vi "Attach Panel Thread.vi"(8 "error in (no error)":errorcluster, 10 "Panel Thread":refnum<class "Panel Controller Interface.lvclass">, 11 "Panel Manager Controller.lvclass":refnum<class "Panel Manager Controller.lvclass">) -> (0 "error out":errorcluster, 3 "Panel Manager Controller.lvclass out":refnum<class "Panel Manager Controller.lvclass">)   [LabVIEW 2015, in "Panel Manager Controller.lvclass"]
uses:
  Panel Manager Controller.lvclass
  _Depences/Panel API/Panel Control_Interface/Panel_interface/Panel Controller Interface.lvclass
  Panel Manager Controller.lvclass/Panel Manager Controller.ctl
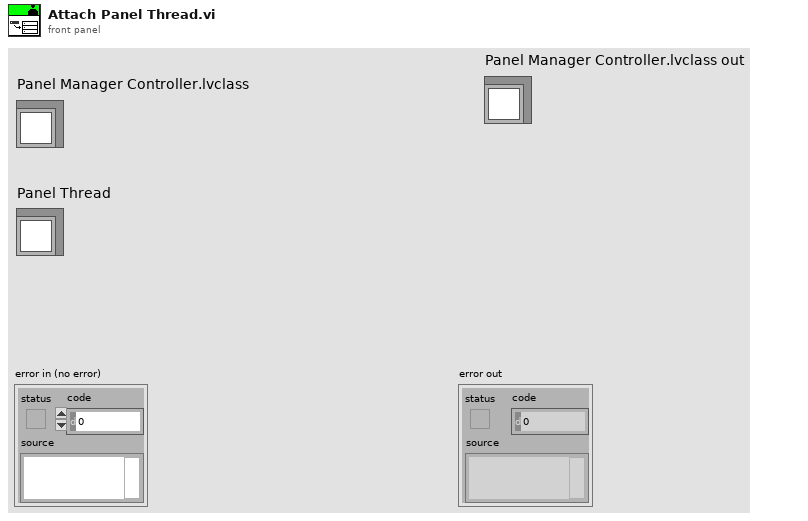
[diagram p1: front panel]
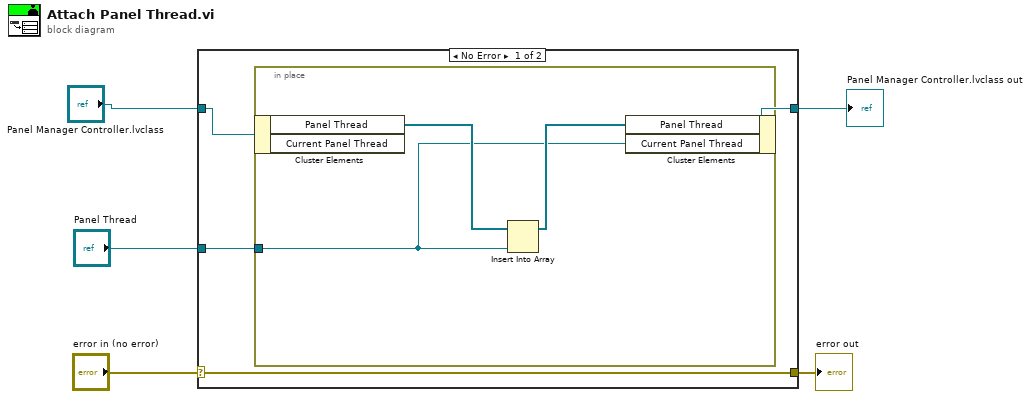
[diagram p0: block diagram]
diagram:
  n1 = case shown="No Error" "error in (no error)" {
    selector: "error in (no error)" -> [w6 w14]
    tunnel: [w6 w14] -> w4
    tunnel: [w7 w13] -> w1
    tunnel: "Panel Manager Controller.lvclass" -> [w9 w13]
    tunnel: "Panel Thread" -> [w8 _]
    frame No Error {
      n2 = in-place {
        in-place-border: w8 -> [w10]
        n3 = in-place-cluster #1(w9) -> ("Panel Thread"=w12:refnum<class "Panel Controller Interface.lvclass">[])  [unwired: 1 out]
        n4 = Insert Into Array(array=w12, new element=w10) -> (w11:refnum<class "Panel Controller Interface.lvclass">[])  [unwired: 1 in]
        n5 = in-place-cluster #1("Panel Thread"=w11, "Current Panel Thread"=w10) -> (w7:refnum<class "Panel Manager Controller.lvclass">)
      }
    }
    frame Error {
    }
  }
  "error out" <- w4
  "Panel Manager Controller.lvclass out" <- w1
